vi "Broadcast.vi"(8 "error in":errorcluster, 10 "myData":dbl) -> (0 "error out":errorcluster)   [LabVIEW 2017, in "SingletonModule.lvlib"]
doc: "Broadcast event method\n_____\nCreated using DQMH Event Scripter 6.1.0.128."
uses:
  SingletonModule.lvlib
  Broadcast Argument--cluster.ctl
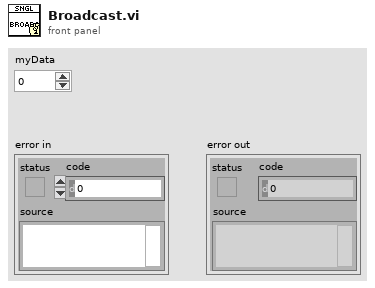
[diagram p1: front panel]
types:
  T1 = typedef "SingletonModule.lvlib/Broadcast Argument--cluster.ctl" = cluster{"myData":dbl}
  T2 = typedef "SingletonModule.lvlib/Broadcast Events--cluster.ctl" = cluster{"Module Did Init":refnum<user-event>, "Status Updated":refnum<user-event>, "Error Reported":refnum<user-event>, "Module Did Stop":refnum<user-event>, "Update Module Execution Status":refnum<user-event>, "Broadcast":refnum<user-event>}
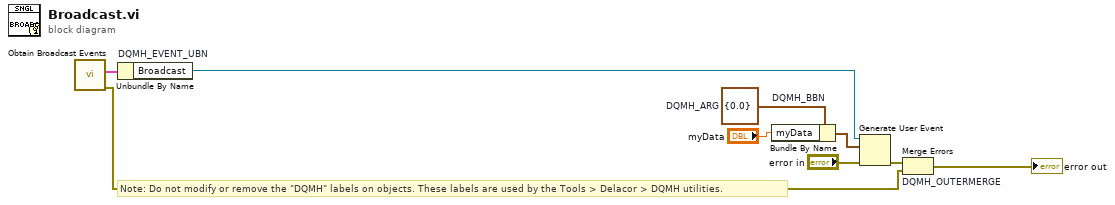
[diagram p0: block diagram]
diagram:
  w4 = T1 {"myData"=0.0}  # DQMH_ARG
  # "Note: Do not modify or remove the \"DQMH\" labels on objects. These labels are used by the Tools > Delacor > DQMH utilities."
  n1 = call "Obtain Broadcast Events.vi"() -> ("error out"=w2:errorcluster, "SingletonModule Broadcast Events"=w1:T2)  [unwired: 10 in]
  n2 = Unbundle By Name "DQMH_EVENT_UBN"(w1) -> ("Broadcast"=w6:refnum<user-event>)
  n3 = Bundle By Name "DQMH_BBN"(cluster=w4, "myData"="myData") -> (w7:T1)
  n4 = Generate User Event(user event=w6, event data cluster=w7, error in="error in") -> (error out=w5:errorcluster)  [unwired: 1 in, 1 out]
  n5 = Merge Errors "DQMH_OUTERMERGE"(w5, w2) -> (→"error out":errorcluster)
